vi "SVPO Power Spectrum (1 Ch DBL WDT).vi"(0 "scaled signal [EU]":waveform(dbl), 2 "window":T7=1 items=["None"=0, "Hanning"=1, "Hamming"=2, "Blackman-Harris"=3, "Exact Blackman"=4, "Blackman"=5, "Flat Top"=6, "4 Term B-Harris "=7, "7 Term B-Harris"=8, "Low Sidelobe"=9, "Force"=64, "Exponential"=65, "Blackman Nuttall"=11, "Triangle"=30, "Bartlett-Hanning"=31, "Bohman"=32, "Parzen"=33, "Welch"=34, "Kaiser"=60, "Dolph-Chebyshev"=61, "Gaussian"=62], 9 "restart averaging? (F)":bool) -> (13 "averages completed":dbl, 14 "power spectrum [EU^2 rms]":cluster{"f0":dbl, "df":dbl, "magnitude":dbl[]} {"magnitude" format="%.2p"; "df" format="%.2p"; "f0" format="%.2p"}, 18 "spectrum info":T1={"channel name"="", "description"="", "x-axis units"=0, "spectral info"={"spectrum type"=enum."Power [Magnitude^2]", "linear/dB"=enum."linear", "window"=0, "window size"=0, "FFT size"=0}, "engineering units"=0, "custom label"="", "dB reference [EU]"=0.0, "peak units"=enum."rms", "weighting filter"=0, "spectral density?"=FALSE, "unit label"="", "spectrum skewed?"=FALSE, "complimentary spectrum units"=enum."none"} {"x-axis units" items=["Time (s)"=0, "Frequency-CB (Hz)"=1, "Frequency-CPB (Hz)"=1248, "Frequency-Arbitrary (Hz)"=2357, "Quefrency (s)"=2, "Revolutions (rev)"=3, "Order"=4, "Speed (RPM)"=11, "Speed (rad/s)"=21, "Index"=65535]; "weighting filter" items=["Linear", "A-weighting", "B-weighting", "C-weighting", "ITU-R 468-4", "Dolby", "CCITT", "C-message", "Wb", "Wc", "Wd", "We", "Wf", "Wh", "Wj", "Wk", "Wm", "AES17 20 kHz lowpass", "AES17 40 kHz lowpass", "AES17 20 kHz highpass", "AES17 40 kHz highpass"]; "dB reference [EU]" format="%.2f"; "engineering units" items=["custom..."=0, "V"=1, "A"=21, "C"=30, "pC"=31, "s"=32, "-"=29, "Pa"=2, "N"=20, "g"=3, "m/s^2"=4, "m/s"=5, "m"=6, "mm/s"=12, "mm"=13, "micron/s"=14, "micron"=15, "in/s^2"=7, "in/s"=8, "in"=9, "mil/s"=10, "mil"=11, "rad/s^2"=16, "rad/s"=17, "rad"=18, "deg/s^2"=26, "deg/s"=27, "deg"=28, "RPM"=22, "cycle/s^2"=23, "Hz"=24, "cycle"=25, "strain"=19]; "spectral info"."window" items=["None "=0, "Hanning"=1, "Hamming"=2, "Blackman-Harris"=3, "Exact Blackman"=4, "Blackman"=5, "Flat Top"=6, "4 Term B-Harris "=7, "7 Term B-Harris"=8, "Low Sidelobe"=9, "Force - Exponential"=10, "Gaussian"=62]})   [LabVIEW 2017]
doc: "Computes the linear RMS-averaged power spectrum of <B>scaled signal [EU]</B> in a linear scale. Use the power spectrum to quantify signal components as a function of frequency. Use this VI on embedded targets that have limited computational resources. Wire data to the <B>scaled signal [EU]</B> input to determine the polymorphic instance to use or manually select the instance."
uses:
  <vilib>/addons/_NISVFA/_Shared subVIs/Controls/svc_Window.ctl
  <vilib>/addons/_NISVFA/_Shared subVIs/Controls/svc_Spectrum Info.ctl
  <vilib>/addons/_NISVFA/_Shared subVIs/Controls/svc_X-Axis Units.ctl
  <vilib>/addons/_NISVFA/_Shared subVIs/Controls/svc_Spectrum Type.ctl
  <vilib>/addons/_NISVFA/_Shared subVIs/Controls/svc_Engineering Units Text Ring.ctl
  <vilib>/addons/_NISVFA/_Shared subVIs/Controls/svc_Weighting Filter Text Ring.ctl
  <vilib>/addons/_NISVFA/_Shared subVIs/Controls/svc_Complimentary Spectrum Units.ctl
  <vilib>/Analysis/2dsp.llb/Power Spectrum (DBL).vi
  <vilib>/Analysis/4window.llb/Force Window.vi
  <vilib>/Analysis/4window.llb/Force Window (DBL).vi
  <vilib>/Analysis/4window.llb/Exponential Window.vi
  <vilib>/Analysis/4window.llb/Exponential Window (DBL).vi
  <vilib>/Utility/error.llb/Error Cluster From Error Code.vi
  <vilib>/Analysis/0measdsp.llb/Scaled Time Domain Window.vi
  <vilib>/Analysis/0measdsp.llb/Scaled Time Domain Window (DBL).vi
  <vilib>/addons/_NISVFA/_Spectrum Processing/subVIs/svfa_Spectrum Info Window to windowTd Type Def.vi
  <vilib>/Analysis/NI_AALPro.lvlib
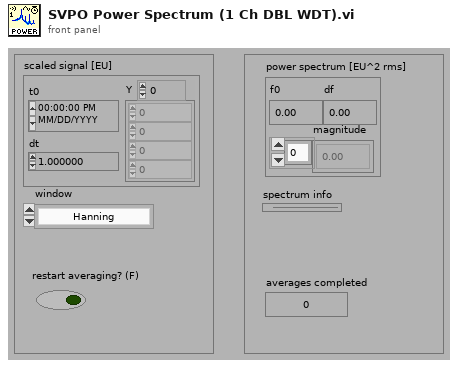
[diagram p1: front panel]
types:
  T1 = typedef "svc_Spectrum Info.ctl" = cluster{"channel name":string, "description":string, "x-axis units":T2, "spectral info":cluster{"spectrum type":T3, "linear/dB":enum16{"linear", "dB"}, "window":u16, "window size":i32, "FFT size":i32}, "engineering units":T4, "custom label":string, "dB reference [EU]":dbl, "peak units":enum16{"rms", "peak", "peak-peak"}, "weighting filter":T5, "spectral density?":bool, "unit label":string, "spectrum skewed?":bool, "complimentary spectrum units":T6}
  T2 = typedef "svc_X-Axis Units.ctl" = u16
  T3 = typedef "svc_Spectrum Type.ctl" = enum16{"FFT Spectrum [complex]", "Amplitude [Magnitude]", "Power [Magnitude^2]", "Cross Spectrum [complex]", "Frequency Response [Complex]"}
  T4 = typedef "svc_Engineering Units Text Ring.ctl" = u16
  T5 = typedef "svc_Weighting Filter Text Ring.ctl" = u16
  T6 = typedef "svc_Complimentary Spectrum Units.ctl" = enum16{"none", "radians", "degrees", "cycles", "imaginary"}
  T7 = typedef "svc_Window.ctl" = u32
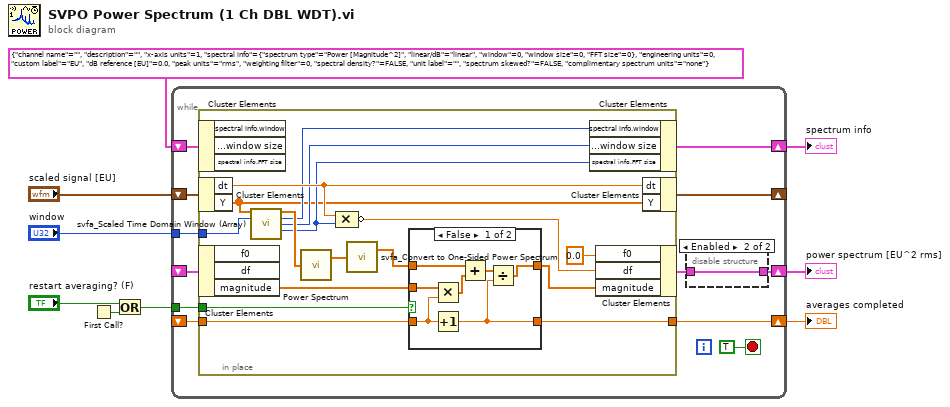
[diagram p0: block diagram]
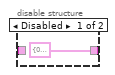
[diagram p2: hidden frame]
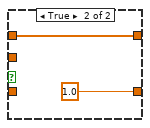
[diagram p3: hidden frame]
diagram:
  n1 = First Call?() -> (First Call?: T/F=w5:bool)
  n2 = Or(x="restart averaging? (F)", y=w5) -> (x .or. y?=w4:bool)
  n3 = while {
    tunnel: "window" -> [w20]
    tunnel: w4 -> [w12]
    shift-right: [w13] -> w1
    shift-left: _ -> [w15]
    shift-right: [w10] -> w2
    shift-left: _ -> [w11]
    shift-right: [w17] -> w7
    shift-left: T1 {"channel name"="", "description"="", "x-axis units"=1, "spectral info"={"spectrum type"=enum."Power [Magnitude^2]", "linear/dB"=enum."linear", "window"=0, "window size"=0, "FFT size"=0}, "engineering units"=0, "custom label"="EU", "dB reference [EU]"=0.0, "peak units"=enum."rms", "weighting filter"=0, "spectral density?"=FALSE, "unit label"="", "spectrum skewed?"=FALSE, "complimentary spectrum units"=enum."none"} ("spectrum info in") -> [w18]
    shift-right: [w16] -> _
    shift-left: "scaled signal [EU]" -> [w19]
    stop <- TRUE stop-if-true
    n4 = in-place {
      in-place-border: w20 -> [w28]
      in-place-border: w12 -> [w31]
      in-place-border: w11 -> [w30]
      in-place-border: [w29] -> w10
      n5 = in-place-cluster #1(w18) -> ()  [unwired: 3 out]
      n6 = in-place-cluster #2(w19) -> ("dt"=w38:dbl, "Y"=w24:dbl[])
      n7 = in-place-cluster #3(w15) -> ("magnitude"=w32:dbl[])  [unwired: 2 out]
      n8 = call <vilib>:"svfa_Scaled Time Domain Window (Array).vi"("input signal"=w24, "window"=w28) -> ("windowed signal"=w37:dbl[], "dup window"=w27:T7, "window length"=w26:i32, "FFT length"=w25:i32)  [unwired: 8 in, 2 out]
      n9 = call-poly <vilib>:"Power Spectrum.vi"("X"=w37) -> ("Power Spectrum"=w39:dbl[])  [unwired: 1 out]
      n10 = Compound Arithmetic op=MULTIPLY(w38, w25) -> (invert w34:dbl)
      n11 = call <vilib>:"svfa_Convert to One-Sided Power Spectrum.vi"("two-sided power spectrum"=w39) -> ("one-sided power spectrum"=w33:dbl[])  [unwired: 1 out]
      n12 = case shown="False" w31 {
        tunnel: [w46 w48] -> w36
        tunnel: [w45 1.0 ("t")] -> w29
        tunnel: w33 -> [w44 w48]
        tunnel: w30 -> [w41 _]
        tunnel: w32 -> [w40 _]
        frame False {
          n13 = Multiply(x=w40, y=w41) -> (x*y=w43:dbl[])
          n14 = Increment(x=w41) -> (x+1=w45:dbl)
          n15 = Add(x=w44, y=w43) -> (x+y=w42:dbl[])
          n16 = Divide(x=w42, y=w45) -> (x/y=w46:dbl[])
        }
        frame True {
        }
      }
      n17 = in-place-cluster #1("spectral info.window"=w27, "spectral info.window size"=w26, "spectral info.FFT size"=w25) -> (w17:T1)
      n18 = in-place-cluster #3("f0"=0.0, "df"=w34, "magnitude"=w36) -> (w14:cluster{"f0":dbl, "df":dbl, "magnitude":dbl[]})
      n19 = in-place-cluster #2("dt"=w38, "Y"=w24) -> (w16:waveform(dbl))
    }
    n20 = disable-structure shown="Enabled" {
      disable-tunnel: [cluster{"f0":dbl, "df":dbl, "magnitude":dbl[]} {"f0"=0.0, "df"=0.0, "magnitude"=[]} ("power spectrum [EU] 2") w23] -> w13
      disable-tunnel: w14 -> [_ w23]
      frame Disabled {
      }
      frame Enabled {
      }
    }
  }
  "power spectrum [EU^2 rms]" <- w1
  "spectrum info" <- w7
  "averages completed" <- w2
